vi "Set Expected.vi"(10 "CANopen Message":refnum<class "CANopen Response Message.lvclass">, 11 "SDO Response Compare Strategy in":refnum<class "SDO Response Compare Strategy.lvclass">) -> (3 "SDO Response Compare Strategy out":refnum<class "SDO Response Compare Strategy.lvclass">)   [LabVIEW 2024, in "CANopen Master.lvlib" / "SDO Response Compare Strategy.lvclass"]
uses:
  SDO Response Compare Strategy.lvclass
  SDO Response Compare Strategy.lvclass/SDO Response Compare Strategy.ctl
  CANopen Response/CANopen Response Message.lvclass
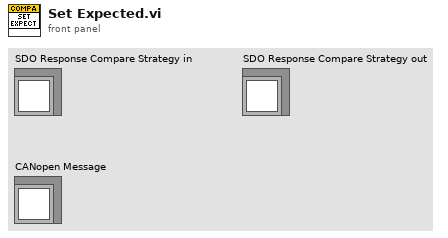
[diagram p1: front panel]
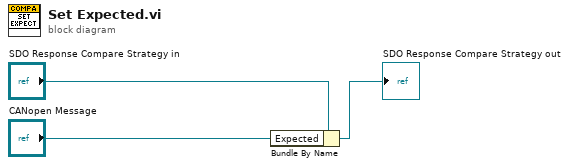
[diagram p0: block diagram]
diagram:
  n1 = Bundle By Name(cluster="SDO Response Compare Strategy in", "Expected"="CANopen Message") -> (→"SDO Response Compare Strategy out":refnum<class "SDO Response Compare Strategy.lvclass">)
